vi "test1.vi"() -> ()   [LabVIEW 2013]
uses:
  <vilib>/LabVIEW Interface for Arduino/Type Defs/Board Type.ctl
  <vilib>/LabVIEW Interface for Arduino/Type Defs/Connection Type.ctl
  <vilib>/LabVIEW Interface for Arduino/Type Defs/Pin Mode.ctl
  <vilib>/LabVIEW Interface for Arduino/LabVIEW Interface for Arduino.lvlib
  <vilib>/measure/NI_MABase.lvlib
panel:
  out "Numeric":dbl
  out "Boolean":bool
  in  "milliseconds to wait":u32
  in  "offset":dbl format="%0.2p"
  in  "stop":bool
  out "Waveform Chart":waveform(dbl)(graph)
  in  "duty cycle (%)":dbl=50.0 format="%0.2f"
  in  "phase":dbl format="%.2p"
  in  "amplitude":dbl=1.0 format="%0.2p"
  in  "frequency":dbl=10.0 format="%0.2p"
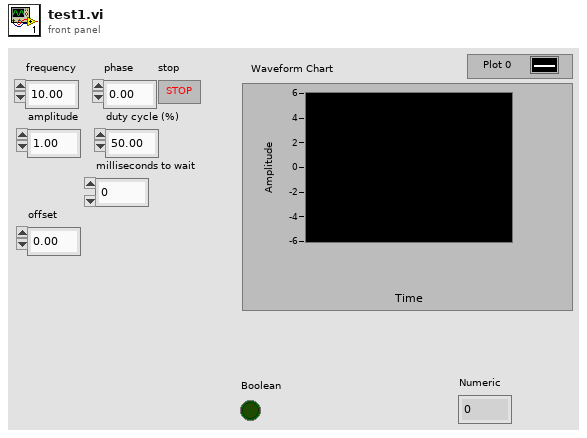
[diagram p1: front panel]
types:
  T1 = typedef "LabVIEW Interface for Arduino.lvlib/Connection Type.ctl" = enum8{"USB / Serial", "XBEE", "BlueSmirf (Bluetooth)"}
  T2 = typedef "LabVIEW Interface for Arduino.lvlib/Board Type.ctl" = enum16{"Uno", "Dimuelanove w/Atmega 328", "Mega 2560"}
  T3 = typedef "LabVIEW Interface for Arduino.lvlib/Arduino Resource.ctl" = cluster{"VISA resource":refnum<visa-resource-name>, "Board Type":T2, "Connection Type":enum8{"USB / Serial"}, "Bytes Per Packet (15)":u8}
  T4 = typedef "LabVIEW Interface for Arduino.lvlib/Pin Mode.ctl" = enum8{"Input", "Output"}
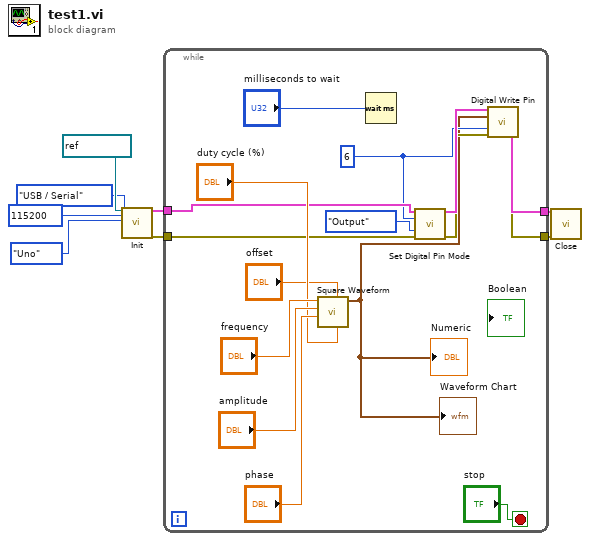
[diagram p0: block diagram]
diagram:
  n1 = call <vilib>:"Init.vi"("VISA resource"=refnum<visa-resource-name> "COM5", "Baud Rate (115200)"=u32 115200, "Board Type (Uno)"=Board_Type."Uno", "Connection Type (USB/Serial)"=Connection_Type."USB / Serial") -> ("Arduino Resource"=w6:T3, "error out"=w5:errorcluster)  [unwired: 14 in]
  n2 = while {
    tunnel: [w17] -> w8
    tunnel: [w16] -> w7
    tunnel: w6 -> [w14]
    tunnel: w5 -> [w13]
    stop <- "stop" stop-if-true
    w11 = u8 6 ("Digital I/O Pin")
    n3 = call <vilib>:"Square Waveform.vi"("duty cycle (%)"="duty cycle (%)", "offset"="offset", "phase"="phase", "amplitude"="amplitude", "frequency"="frequency") -> ("signal out"=w9:waveform(dbl))  [unwired: 5 in, 1 out]
    "Waveform Chart" <- w9
    "Numeric" <- w9
    n4 = Wait (ms)(milliseconds to wait="milliseconds to wait") -> ()  [unwired: 1 out]
    n5 = call <vilib>:"Set Digital Pin Mode.vi"("Arduino Resource"=w14, "Digital I/O Pin"=w11, "Pin Mode (Input)"=Pin_Mode."Output", "error in"=w13) -> ("Arduino Resource"=w18:T3, "error out"=w15:errorcluster)  [unwired: 10 in]
    n6 = call <vilib>:"Digital Write Pin.vi"("Arduino Resource"=w18, "Digital I/O Pin (0)"=w9, "Value (0)"=w11, "error in"=w15) -> ("Arduino Resource"=w17:T3, "error out"=w16:errorcluster)  [unwired: 10 in]
  }
  n7 = call <vilib>:"Close.vi"("Arduino Resource"=w8, "error in"=w7) -> ()  [unwired: 13 in, 1 out]
